vi "Nxt name.vi"(0 "Full string":string, 1 "MAX":i32, 2 "Seq":i32) -> (3 "general TP info":string, 4 "Nxt.Name":string[](array[string]), 5 "tpdata":string[](array[string]), 6 "Ext.Name string":string)   [LabVIEW 2018]
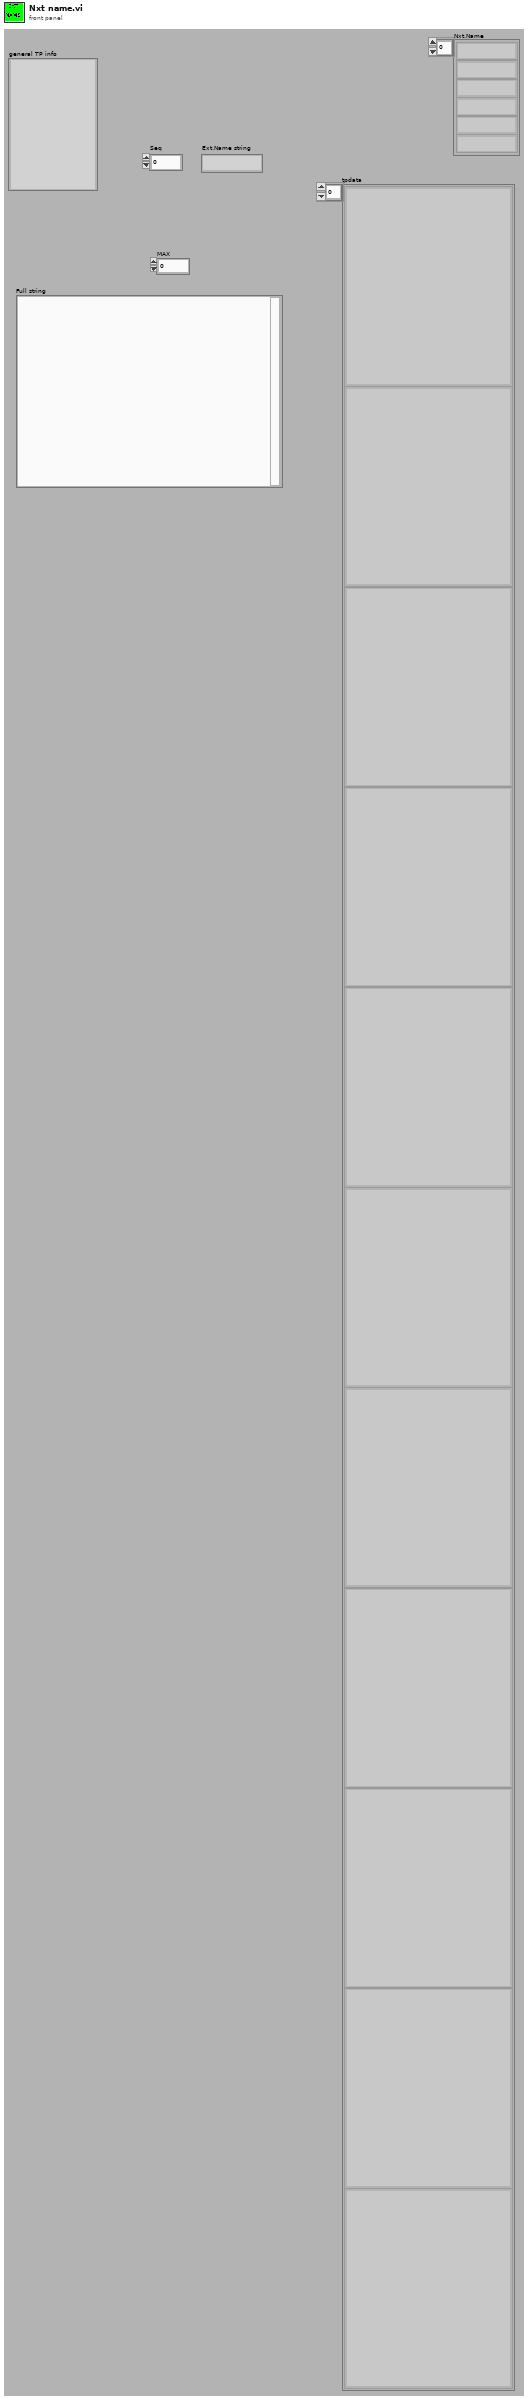
[diagram p1: front panel]
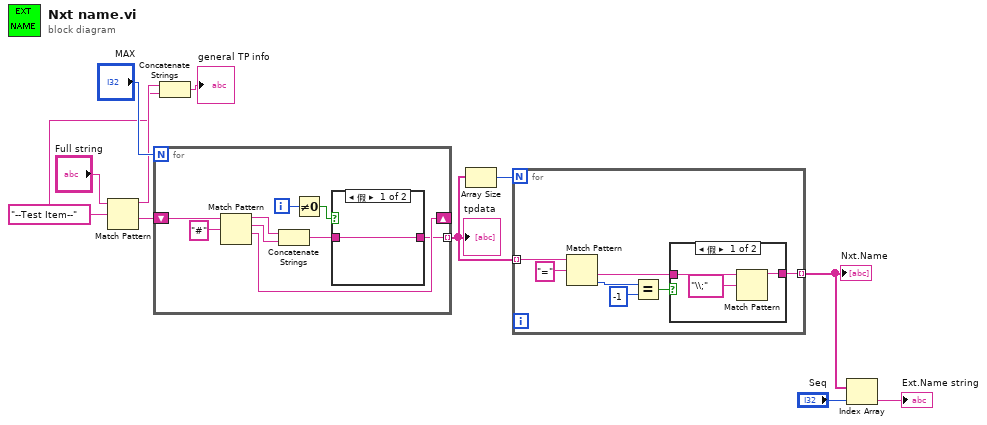
[diagram p0: block diagram]
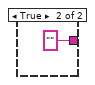
[diagram p2: hidden frame]
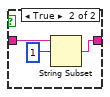
[diagram p3: hidden frame]
diagram:
  w1 = "--Test Item--" ("regular expression")
  n1 = Match Pattern(string="Full string", regular expression=w1) -> (before substring=w3:string, after substring=w9:string)  [unwired: 3 out]
  n2 = for {
    N: "MAX" -> [_]
    shift-right: [w18] -> _
    shift-left: w9 -> [w20]
    tunnel: [w12] -> w8 mode=indexing
    i -> [w15]
    n3 = Match Pattern(string=w20, regular expression="#") -> (before substring=w17:string, match substring=w16:string, after substring=w18:string)  [unwired: 2 out]
    n4 = Concatenate Strings(w17, w16) -> (w13:string)
    n5 = Not Equal To 0?(x=w15) -> (x != 0?=w14:bool)
    n6 = case shown="假" w14 {
      tunnel: w13 -> [w21 w23]
      tunnel: [w21 w22] -> w12
      frame False {
      }
      frame True {
        n7 = String Subset(string=w23, offset (0)=1 ("偏移量(0)")) -> (substring=w22:string)  [unwired: 1 out]
      }
    }
  }
  "tpdata" <- w8
  n8 = Concatenate Strings(w3, w1) -> (→"general TP info":string)
  n9 = Array Size(array=w8) -> (size(s)=w7:i32)
  n10 = for {
    N: w7 -> [_]
    tunnel: w8 -> [w31] mode=indexing
    tunnel: [w25] -> w6 mode=indexing
    n11 = Match Pattern(string=w31, regular expression="=") -> (after substring=w26:string, offset past match=w29:i32)  [unwired: 3 out]
    n12 = Equal?(x=w29, y=-1) -> (x = y?=w27:bool)
    n13 = case shown="假" w27 {
      tunnel: [w32 ""] -> w25
      tunnel: w26 -> [w34 _]
      frame False {
        n14 = Match Pattern(string=w34, regular expression="\\;") -> (before substring=w32:string)  [unwired: 4 out]
      }
      frame True {
      }
    }
  }
  "Nxt.Name" <- w6
  n15 = Index Array(array=w6, index="Seq") -> (element=→"Ext.Name string":string)
